vi "lab3a.vi"() -> ()   [LabVIEW 2019]
uses:
  <vilib>/Platform/TimedLoop/XDataNode/timing_clust.ctl
  <vilib>/Platform/TimedLoop/XDataNode/nitl_modes.ctl
  <vilib>/Platform/TimedLoop/XDataNode/wakeup.ctl
  <vilib>/Analysis/3filter.llb/Filter Passband Type.ctl
  <vilib>/DAQmx/write.llb/DAQmx Write (Analog DBL 1Chan 1Samp).vi
  <vilib>/DAQmx/read.llb/DAQmx Read (Analog DBL 1Chan 1Samp).vi
  <vilib>/DAQmx/create/channels.llb/DAQmx Create Channel (AO-Voltage-Basic).vi
  <vilib>/DAQmx/miscellaneous.llb/DAQmx Fill In Error Info.vi
  <vilib>/DAQmx/create/channels.llb/DAQmx Create Channel (AI-Voltage-Basic).vi
  <vilib>/platform/TimedLoop/XDataNode/XDataNode.xnode
  <vilib>/Platform/TimedLoop/XDataNode/XDNodeRunTimeDep.lvlib
  <vilib>/ptbypt/NI_PtbyPt.lvlib
  <vilib>/Analysis/NI_AALBase.lvlib
panel:
  out "Position":dbl(graph)
  out "Position":dbl
  out "Position":dbl(knob) scale=-32.5..32.5
  out "Voltage":dbl(graph)
  in  "stop":bool
  in  "low cutoff freq: Position":dbl=0.125 format="%0.3f"
  in  "Amplitude":dbl
  in  "Frequency":dbl
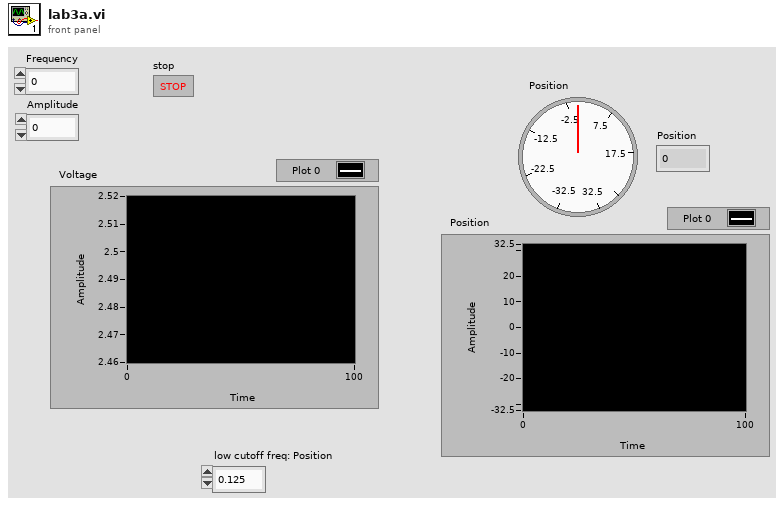
[diagram p1: front panel]
types:
  T1 = typedef "NI_AALBase.lvlib/Filter Passband Type.ctl" = enum32{"Lowpass", "Highpass", "Bandpass", "Bandstop"}
  T2 = typedef "XDNodeRunTimeDep.lvlib/timing_clust.ctl" = cluster{"Expected End [f-1]":u64, "Actual End [f-1]":u64, "Finished Late? [f-1]":bool, "Expected End [i-1]":u64, "Actual End [i-1]":u64, "Finished Late? [i-1]":bool, "Expected Start [i]":u64, "Actual Start [i]":u64, "Expected Start [f]":u64, "Actual Start [f]":u64, "Source Name":string, "Structure Name":string, "Period":i64, "Deadline":i64, "Offset":i64, "Start":i64, "Priority":i32, "Timeout":i32, "Mode":T3, "Wakeup Reason":T4, "Error":errorcluster, "Source Type":string, "Secondary Source Type":string, "Global End Time":u64, "Global Start Time":u64, "Frame Duration":u64, "Iteration Duration":u64, "Assigned CPU":i32, "I/O Scan Engine Mode":u32}
  T3 = typedef "XDNodeRunTimeDep.lvlib/nitl_modes.ctl" = enum32{"No Change", "Process missed periods, maintain original phase", "Discard missed periods, maintain original phase", "Process missed periods, ignore original phase", "Discard missed periods, ignore original phase"}
  T4 = typedef "XDNodeRunTimeDep.lvlib/wakeup.ctl" = enum32{"Normal", "Aborted", "Asynchronous wakeup", "Timing source error", "Timed loop error", "Timeout"}
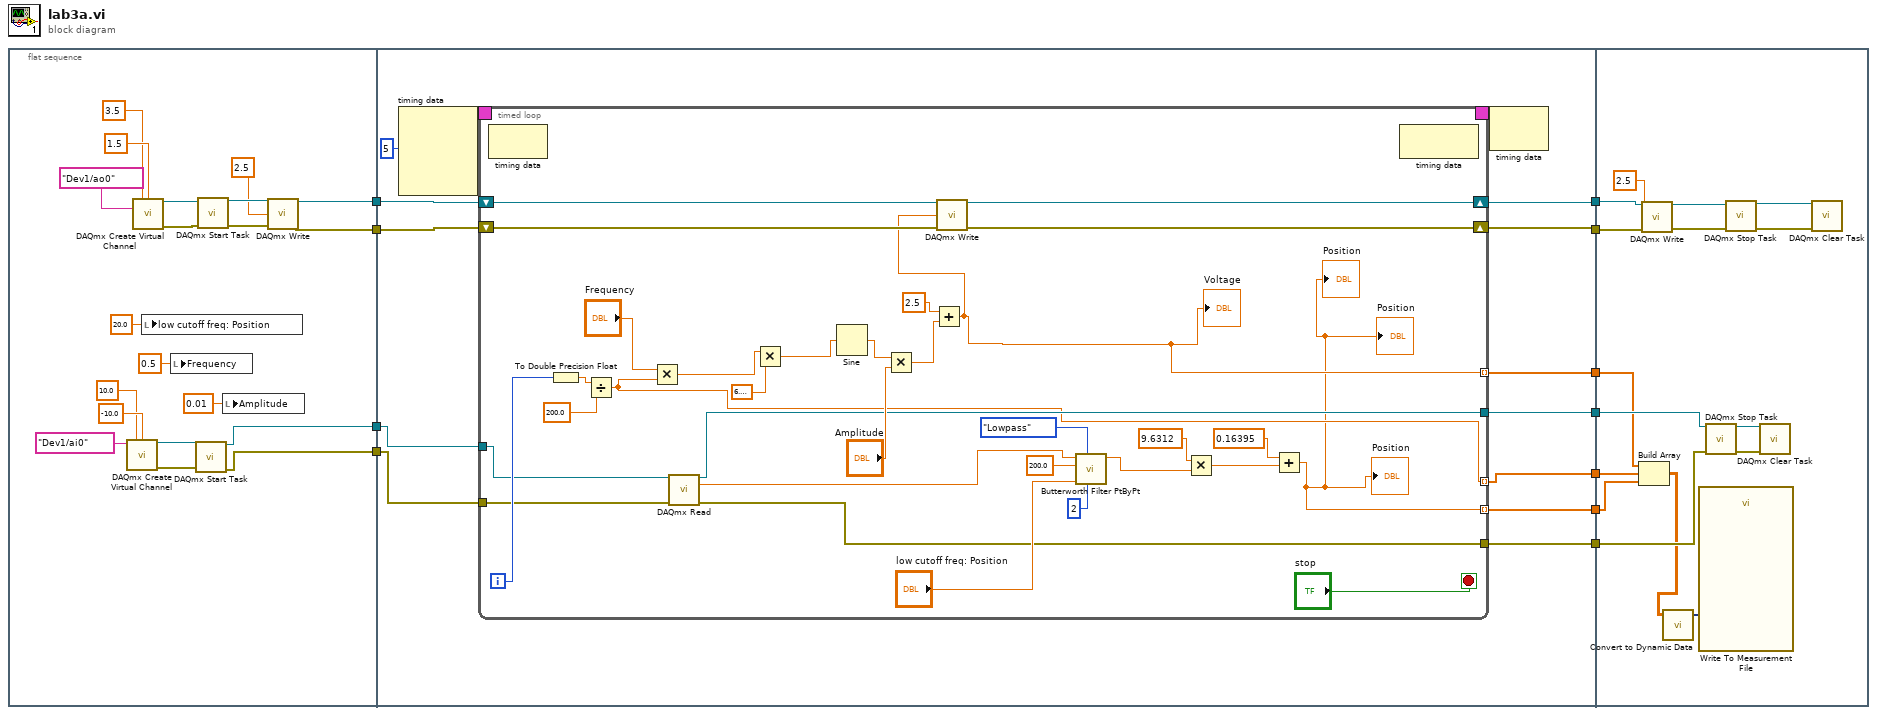
[diagram p0: block diagram]
diagram:
  n1 = flat-sequence {
    tunnel: [w29] -> w11
    tunnel: [w28] -> w10
    tunnel: [w16] -> w9
    tunnel: [w15] -> w8
    tunnel: w11 -> [w45]
    tunnel: w10 -> [w43]
    tunnel: w9 -> [w38]
    tunnel: w8 -> [w37]
    tunnel: [w44] -> w7
    tunnel: [w42] -> w6
    tunnel: [w36] -> w5
    tunnel: [w35] -> w4
    tunnel: [w34] -> w3
    tunnel: [w33] -> w2
    tunnel: [w32] -> w1
    tunnel: w7 -> [w91]
    tunnel: w6 -> [w90]
    tunnel: w5 -> [w89]
    tunnel: w4 -> [w88]
    tunnel: w3 -> [w87]
    tunnel: w2 -> [w86]
    tunnel: w1 -> [w84]
    frame #0 {
      n2 = call-poly <vilib>:"DAQmx Create Virtual Channel.vi"("maximum value"=10.0, "minimum value"=-10.0, "physical channels"=tag "Dev1/ai0") -> ("task out"=w21:refnum<k21>, "error out"=w20:errorcluster)  [unwired: 11 in]
      n3 = call-poly <vilib>:"DAQmx Create Virtual Channel.vi"("maximum value"=3.5, "minimum value"=1.5, "physical channels"=tag "Dev1/ao0") -> ("task out"=w31:refnum<k21>, "error out"=w27:errorcluster)  [unwired: 11 in]
      n4 = local write "low cutoff freq: Position"(20.0 ("low cutoff freq: Position")) -> ()
      n5 = local write "Frequency"(0.5 ("Frequency")) -> ()
      n6 = call <vilib>:"DAQmx Start Task.vi"("task/channels in"=w21, "error in"=w20) -> ("task out"=w16:refnum<k21>, "error out"=w15:errorcluster)  [unwired: 12 in]
      n7 = call <vilib>:"DAQmx Start Task.vi"("task/channels in"=w31, "error in"=w27) -> ("task out"=w30:refnum<k21>, "error out"=w26:errorcluster)  [unwired: 12 in]
      n8 = local write "Amplitude"(0.01 ("Amplitude")) -> ()
      n9 = call-poly <vilib>:"DAQmx Write.vi"("task/channels in"=w30, "data"=2.5, "error in"=w26) -> ("task out"=w29:refnum<k21>, "error out"=w28:errorcluster)  [unwired: 10 in, 1 out]
    }
    frame #1 {
      n10 = node-c288(i64 5 ("Period")) -> (w41:T2)  [unwired: 3 in]
      n11 = timed-loop {
        timing: w41 -> [_]
        timing-out: [_] -> w40
        shift-right: [w76] -> w44
        shift-left: w45 -> [w77]
        shift-right: [w74] -> w42
        shift-left: w43 -> [w75]
        tunnel: w38 -> [w67]
        tunnel: w37 -> [w66]
        tunnel: [w56] -> w36
        tunnel: [w55] -> w35
        tunnel: [w50] -> w34 mode=indexing
        tunnel: [w46] -> w33 mode=indexing
        tunnel: [w47] -> w32 mode=indexing
        i -> [w73]
        stop <- "stop" stop-if-true
        n12 = node-c288() -> ()  [unwired: 1 in, 1 out]
        n13 = To Double Precision Float(number=w73) -> (double precision float=w53:dbl)
        n14 = Divide(x=w53, y=200.0) -> (x/y=w50:dbl)
        n15 = Multiply(x="Frequency", y=w50) -> (x*y=w71:dbl)
        n16 = call-poly <vilib>:"DAQmx Read.vi"("task/channels in"=w67, "error in"=w66) -> ("task out"=w56:refnum<k21>, "data"=w57:dbl, "error out"=w55:errorcluster)  [unwired: 11 in]
        n17 = Multiply(x=w71, y=6.283185307179586) -> (x*y=w70:dbl)
        n18 = Sine(x=w70) -> (sin(x)=w68:dbl)
        n19 = Multiply(x=w68, y="Amplitude") -> (x*y=w49:dbl)
        n20 = Add(x=2.5, y=w49) -> (x+y=w47:dbl)
        "Voltage" <- w47
        n21 = call-poly <vilib>:"DAQmx Write.vi"("task/channels in"=w77, "data"=w47, "error in"=w75) -> ("task out"=w76:refnum<k21>, "error out"=w74:errorcluster)  [unwired: 10 in, 1 out]
        n22 = call <vilib>:"Butterworth Filter PtByPt.vi"("order"=2, "filter type"=Filter_Passband_Type."Lowpass", "low cutoff freq: fl"="low cutoff freq: Position", "sampling freq: fs"=200.0, "x"=w57) -> ("Filtered x"=w58:dbl)  [unwired: 4 in, 1 out]
        n23 = Multiply(x=9.6312, y=w58) -> (x*y=w60:dbl)
        n24 = Add(x=0.16395, y=w60) -> (x+y=w46:dbl)
        "Position" <- w46
        "Position" <- w46
        "Position" <- w46
        n25 = node-c288() -> ()  [unwired: 1 in, 1 out]
      }
      n26 = node-c288(w40) -> ()  [unwired: 1 out]
    }
    frame #2 {
      n27 = Build Array(w84, w87, w86) -> (w85:dbl[][])
      n28 = call-poly <vilib>:"DAQmx Write.vi"("task/channels in"=w91, "data"=2.5, "error in"=w90) -> ("task out"=w99:refnum<k21>, "error out"=w96:errorcluster)  [unwired: 10 in, 1 out]
      n29 = call "Convert to Dynamic Data"("2D Array"=w85) -> ("Dynamic Data Type"=w92:dynamicdata)  [unwired: 3 in]
      n30 = call "Write To Measurement File"("Signals"=w92) -> ()  [unwired: 16 in, 3 out]
      n31 = call <vilib>:"DAQmx Stop Task.vi"("task/channels in"=w89, "error in"=w88) -> ("task out"=w94:refnum<k21>, "error out"=w93:errorcluster)  [unwired: 12 in]
      n32 = call <vilib>:"DAQmx Stop Task.vi"("task/channels in"=w99, "error in"=w96) -> ("task out"=w98:refnum<k21>, "error out"=w97:errorcluster)  [unwired: 12 in]
      n33 = call <vilib>:"DAQmx Clear Task.vi"("task in"=w94, "error in"=w93) -> ()  [unwired: 13 in, 1 out]
      n34 = call <vilib>:"DAQmx Clear Task.vi"("task in"=w98, "error in"=w97) -> ()  [unwired: 13 in, 1 out]
    }
  }
